vi "Drive Distance with Vision.vi"(11 "Distance SP":dbl) -> (3 "Done?":bool)   [LabVIEW 2016]
uses:
  Robot Values.vi
  <vilib>/addons/control/pid/pid.llb/PID (DBL).vi
  Vision Global.vi
  <vilib>/addons/control/pid/NI_PID_pid.lvlib
  <vilib>/ptbypt/NI_PtbyPt.lvlib
panel:
  in  "Vision PID Gains":T1={"proportional gain (Kc)"=1.0, "integral time (Ti, min)"=0.01, "derivative time (Td, min)"=0.0} {"derivative time (Td, min)" format="%.3f"; "integral time (Ti, min)" format="%.3f"; "proportional gain (Kc)" format="%.3f"}
  in  "Time Tolerance":dbl=0.15 format="%#_13g"
  out "Elapsed Time (s)":dbl
  in  "Error PID gains":T1={"proportional gain (Kc)"=1.0, "integral time (Ti, min)"=0.01, "derivative time (Td, min)"=0.0} {"derivative time (Td, min)" format="%.3f"; "integral time (Ti, min)" format="%.3f"; "proportional gain (Kc)" format="%.3f"}
  in  "PID gains":T1={"proportional gain (Kc)"=1.0, "integral time (Ti, min)"=0.01, "derivative time (Td, min)"=0.0} {"derivative time (Td, min)" format="%.3f"; "integral time (Ti, min)" format="%.3f"; "proportional gain (Kc)" format="%.3f"}
  # "OLD"
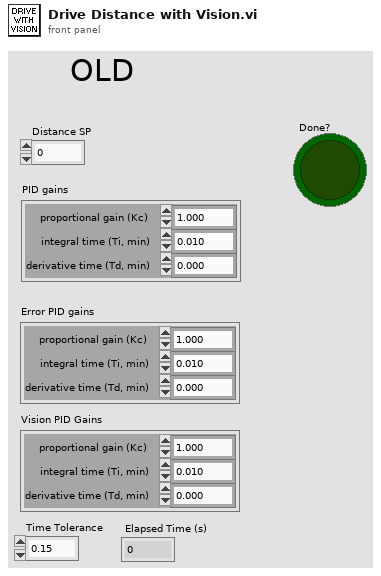
[diagram p1: front panel]
types:
  T1 = cluster{"proportional gain (Kc)":dbl, "integral time (Ti, min)":dbl, "derivative time (Td, min)":dbl}
  T2 = typedef "Robot Values.ctl" = cluster{"Robot Drive":cluster{"Left Motor Power":dbl, "Right Motor Power":dbl, "Left Encoder Value":dbl, "Right Encoder Value":dbl, "High Gear?":bool, "PTO?":bool}, "Sensors":cluster{"Gyro Angle":u16, "Recalibrate Gyro":bool, "Reset Gyro":bool}, "Shooter":cluster{"Prep Wheels":bool, "Shoot":bool, "Left Shooter Wheel Speed":dbl, "Wheels Moving":bool, "Shooter Prepped":bool, "Shooter RPS SP":dbl, "Shooting?":bool, "Left Shooter Wheel Power":dbl, "Right Shooter Wheel Power":dbl, "Acquisition Conveyor Power":dbl, "Hopper Beater Bar Power":dbl, "Filtered Left Shooter Speed":dbl, "Acquisition Motor Power":dbl, "Joystick Add":dbl}, "Robot States":cluster{"Drive mode":string, "Alliance":T3, "Position":T4}, "Gear":cluster{"Ejection Active":bool}}
  T3 = typedef "WPI_DriverStationAllianceInfo.ctl" = enum16{"Red", "Blue", "Invalid"}
  T4 = typedef "WPI_DriverStationPositionInfo.ctl" = enum16{"1", "2", "3"}
  T5 = cluster{"Distance (ft)":dbl, "Score":dbl, "Normalized":cluster{"Center":cluster{dbl, dbl}, "Rectangle":cluster{"Numeric":dbl, "Numeric 2":dbl, "Numeric 3":dbl, "Numeric 5":dbl}}, "Pixels":cluster{"Center":cluster{dbl, dbl}, "Rectangle":cluster{"Numeric":dbl, "Numeric 2":dbl, "Numeric 3":dbl, "Numeric 5":dbl}}}
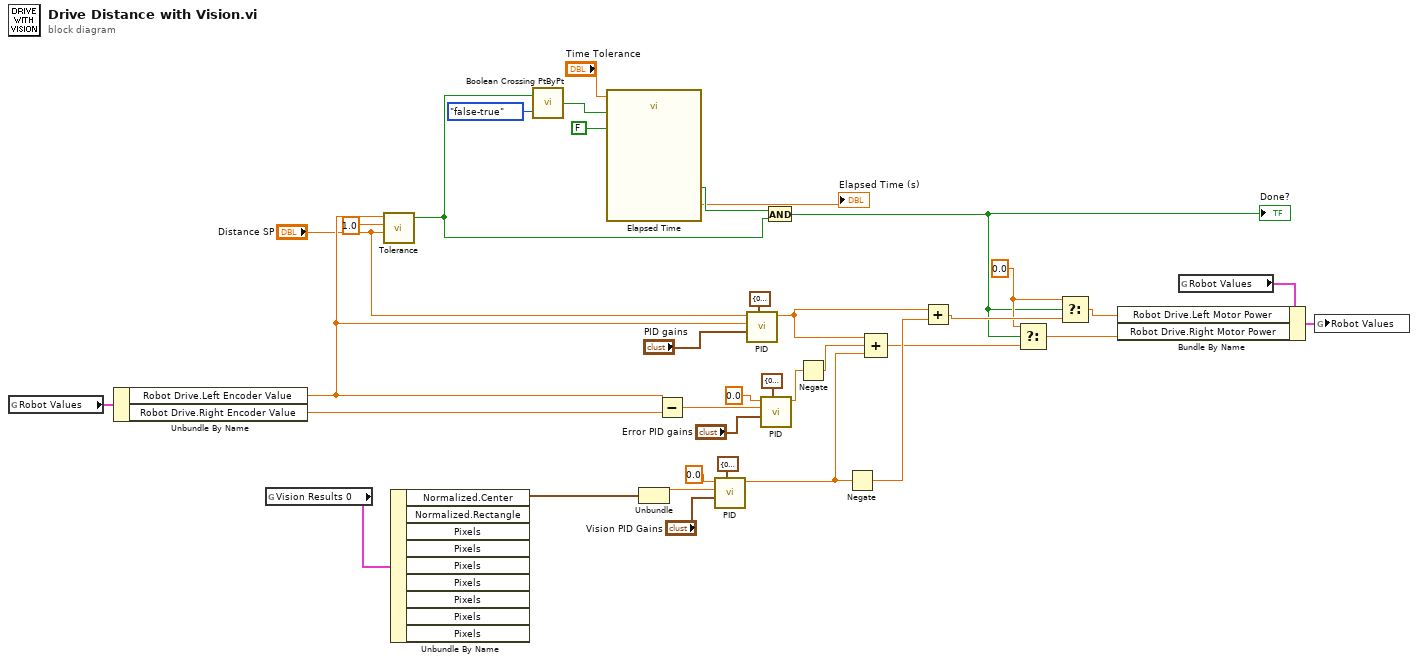
[diagram p0: block diagram]
diagram:
  w3 = 0.0 ("t")
  n1 = global read "Robot Values.vi" "Robot Values"() -> (w37:T2)
  n2 = Unbundle By Name(w37) -> ("Robot Drive.Left Encoder Value"=w25:dbl, "Robot Drive.Right Encoder Value"=w32:dbl)
  n3 = global read "Vision Global.vi" "Vision Results 0"() -> (w15:T5)
  n4 = call "Tolerance.vi"("Setpoint"="Distance SP", "Tolerance"=1.0, "Current Value"=w25) -> ("In Range?"=w16:bool)  [unwired: 8 in]
  n5 = Unbundle By Name(w15) -> ("Normalized.Center"=w14:cluster{dbl, dbl})  [unwired: 8 out]
  n6 = call <vilib>:"Boolean Crossing PtByPt.vi"("direction"=enum16{"either", "false-true", "true-false"}."false-true", "input"=w16) -> ("crossing"=w21:bool)  [unwired: 1 in]
  n7 = call "Elapsed Time"("Time Target (s)"="Time Tolerance", "Reset"=w21, "Auto Reset"=FALSE) -> ("Elapsed Time (s)"=→"Elapsed Time (s)":dbl, "Time has Elapsed"=w18:bool)  [unwired: 9 in, 6 out]
  n8 = Unbundle(w14) -> (w10:dbl)  [unwired: 1 out]
  n9 = Subtract(x=w25, y=w32) -> (x-y=w31:dbl)
  n10 = call-poly <vilib>:"PID.vi"("output range"=cluster{"output high":dbl, "output low":dbl} {"output high"=0.8, "output low"=-0.8}, "PID gains"="Vision PID Gains", "process variable"=w10, "setpoint"=0.0) -> ("output"=w7:dbl)  [unwired: 6 in, 1 out]
  n11 = call-poly <vilib>:"PID.vi"("output range"=cluster{"output high":dbl, "output low":dbl} {"output high"=0.5, "output low"=-0.5}, "PID gains"="PID gains", "process variable"=w25, "setpoint"="Distance SP") -> ("output"=w9:dbl)  [unwired: 6 in, 1 out]
  n12 = call-poly <vilib>:"PID.vi"("output range"=cluster{"output high":dbl, "output low":dbl} {"output high"=0.1, "output low"=-0.1}, "PID gains"="Error PID gains", "process variable"=w31, "setpoint"=0.0) -> ("output"=w27:dbl)  [unwired: 6 in, 1 out]
  n13 = And(x=w18, y=w16) -> (x .and. y?=w2:bool)
  "Done?" <- w2
  n14 = Negate(x=w27) -> (-x=w26:dbl)
  n15 = Negate(x=w7) -> (-x=w8:dbl)
  n16 = Compound Arithmetic op=ADD(w9, w26, w7) -> (w4:dbl)
  n17 = Add(x=w9, y=w8) -> (x+y=w6:dbl)
  n18 = Select(t=w3, s=w2, f=w4) -> (s? t:f=w1:dbl)
  n19 = Select(t=w3, s=w2, f=w6) -> (s? t:f=w5:dbl)
  n20 = global read "Robot Values.vi" "Robot Values"() -> (w33:T2)
  n21 = Bundle By Name(cluster=w33, "Robot Drive.Left Motor Power"=w5, "Robot Drive.Right Motor Power"=w1) -> (w34:T2)
  n22 = global write "Robot Values.vi" "Robot Values"(w34) -> ()
